vi "DevicePortFinder.vi"(3 "Substring":string="LilyPad") -> (0 "Port found":bool, 1 "VISA resource name":refnum<visa-resource-name>)   [LabVIEW 2012]
uses:
  <vilib>/Instr/_visa.llb/VISA Find Search Mode.ctl
  <vilib>/regexp/Match Regular Expression.xnode
panel:
  out "Array":errorcluster[](array[cluster])
  in  "error in (no error) 2":errorcluster
  out "find list 2":string[](array[string])
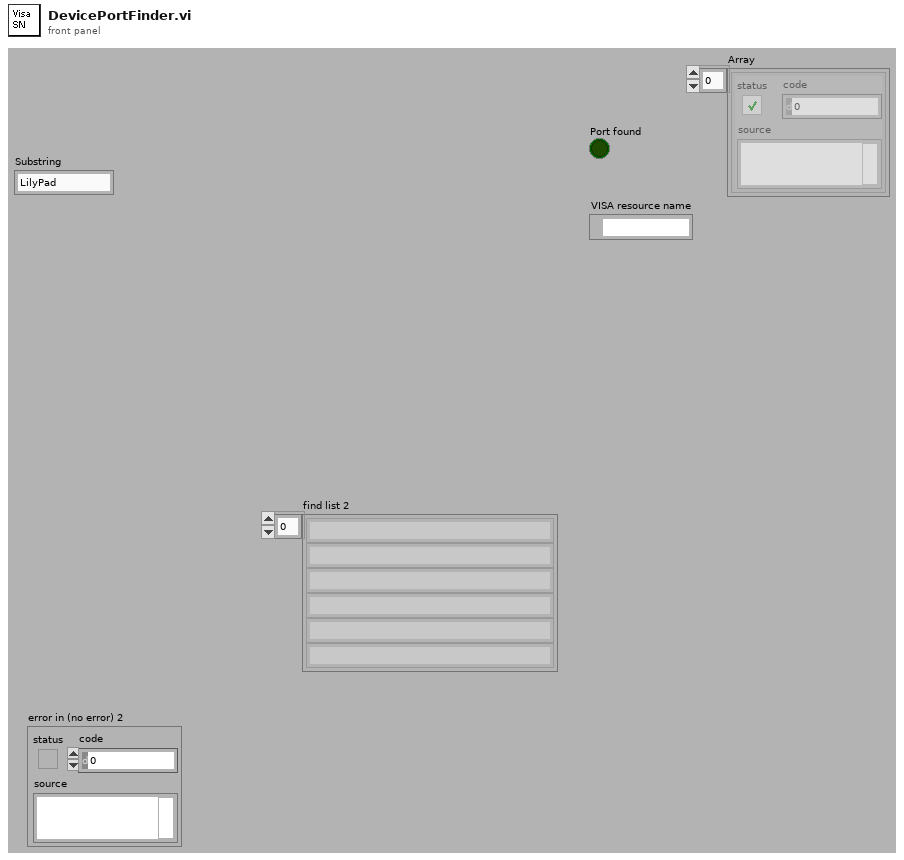
[diagram p1: front panel]
types:
  T1 = typedef "VISA Find Search Mode.ctl" = u32
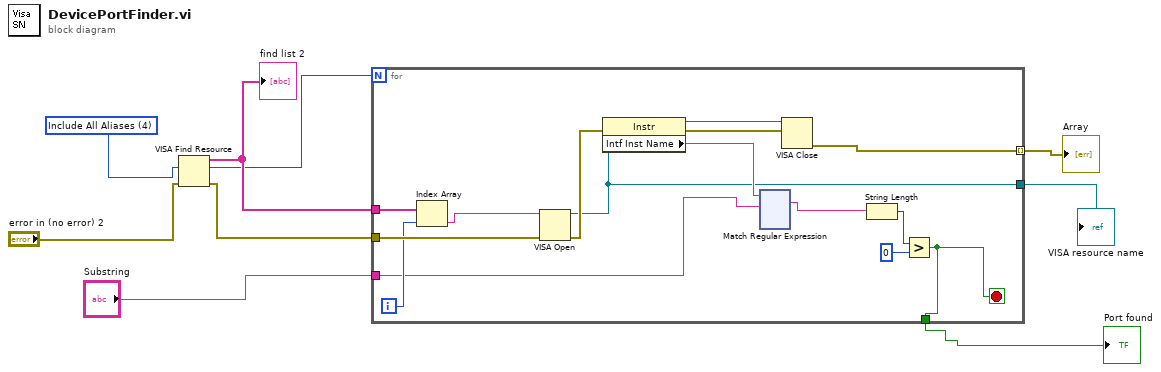
[diagram p0: block diagram]
diagram:
  w9 = T1 4 items=["Canonical Names Only"=0, "Aliases Only"=2, "Include Matching Aliases"=3, "Include All Aliases"=4] ("Search Mode 2")
  n1 = VISA Find Resource(8:"error in (no error) 2", 10:w9) -> (0:w5:errorcluster, 2:w6:u32, 3:w7:string[])  [unwired: 1 in]
  "find list 2" <- w7
  n2 = for {
    N: w6 -> [_]
    tunnel: w7 -> [w21]
    tunnel: w5 -> [w19]
    tunnel: [w18] -> w4 mode=indexing
    tunnel: "Substring" -> [w12]
    tunnel: [w11] -> w2
    tunnel: [w10] -> w1
    i -> [w15]
    stop <- w10 stop-if-true
    n3 = Index Array(array=w21, index=w15) -> (element=w20:string)
    n4 = VISA Open(error in (no error)=w19, VISA resource name=w20) -> (VISA resource name=w11:refnum<visa-resource-name>, error out=w23:errorcluster)  [unwired: 3 in]
    n5 = property class="Instr"(reference=w11, error in=w23) -> (reference out=w22:refnum<visa-resource-name>, error out=w24:errorcluster, "Intf Inst Name"=w14:string)
    n6 = xnode "Match Regular Expression"("input string"=w14, "regular expression"=w12) -> ("whole match"=w13:string)  [unwired: 4 in, 4 out]
    n7 = VISA Close(VISA resource name=w22, error in (no error)=w24) -> (error out=w18:errorcluster)
    n8 = String Length(string=w13) -> (length=w17:i32)
    n9 = Greater?(x=w17, y=0) -> (0:w10:bool)
  }
  "Array" <- w4
  "VISA resource name" <- w2
  "Port found" <- w1
